vi "Array-Find Nearest.vi"(0 "X":dbl[](array[numeric]), 5 "Y":dbl[](array[numeric]), 9 "U":dbl) -> (4 "Xu":dbl, 6 "Yu":dbl, 10 "index":i32)   [LabVIEW 2020]
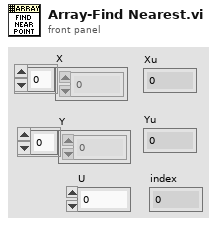
[diagram p1: front panel]
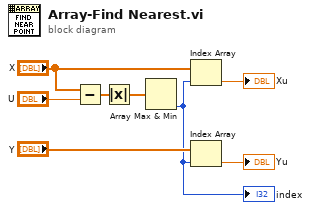
[diagram p0: block diagram]
diagram:
  n1 = Subtract(x="X", y="U") -> (x-y=w7:dbl[])
  n2 = Absolute Value(x=w7) -> (abs(x)=w6:dbl[])
  n3 = Array Max & Min(array=w6) -> (min index (indices)=w2:i32)  [unwired: 3 out]
  "index" <- w2
  n4 = Index Array(array="X", index=w2) -> (element=→"Xu":dbl)
  n5 = Index Array(array="Y", index=w2) -> (element=→"Yu":dbl)
